vi "Read Response to Value Outside Limits.vi"(8 "error in (no error)":errorcluster, 11 "Numeric.lvclass in":refnum<class "Numeric.lvclass">) -> (0 "error out":errorcluster, 2 "RespToValOutLimits":T1, 3 "Numeric.lvclass out":refnum<class "Numeric.lvclass">)   [LabVIEW 2015, in "Numeric.lvclass"]
uses:
  Numeric.lvclass
  <vilib>/Utility/miscctls.llb/LVOutOfRangeActionTypeDef.ctl
  Numeric.lvclass/Numeric.ctl
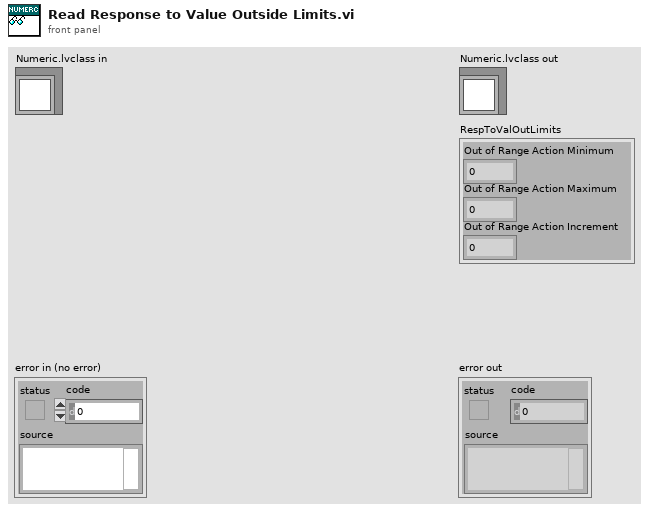
[diagram p1: front panel]
types:
  T1 = typedef "LVOutOfRangeActionTypeDef.ctl" = cluster{"Out of Range Action Minimum":u8, "Out of Range Action Maximum":u8, "Out of Range Action Increment":u8}
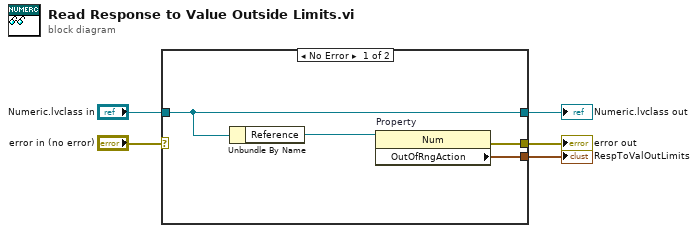
[diagram p0: block diagram]
diagram:
  n1 = case shown="No Error" "error in (no error)" {
    selector: "error in (no error)" -> [_ w11]
    tunnel: [w8 w11] -> w4
    tunnel: [w7 w10] -> w2
    tunnel: "Numeric.lvclass in" -> [w7 w10]
    tunnel: [w9 _] -> w1
    frame No Error {
      n2 = Unbundle By Name(w7) -> ("Reference"=w6:refnum<vi>)
      n3 = property on="Property" class="Num"(reference=w6) -> (error out=w8:errorcluster, "OutOfRngAction"=w9:T1)  [unwired: 1 in, 1 out]
    }
    frame Error {
    }
  }
  "error out" <- w4
  "Numeric.lvclass out" <- w2
  "RespToValOutLimits" <- w1
